vi "BonOMM-SAOMM.Test.vi"() -> ()   [LabVIEW 2011] (continued)
                                n2344 = local write "XReference"(w6163) -> ()
                                n2345 = local write "YReference"(w6164) -> ()
                                n2346 = Multiply(x=15.0, y=w6158) -> (x*y=w6156:dbl)
                                n2347 = Cosine(x=w6151) -> (cos(x)=w6155:dbl)
                                n2348 = Multiply(x=w6155, y=w6156) -> (x*y=w6154:dbl)
                                n2349 = property on="TableXYPos" class="XYGraph (strict)"("Cursor.Cursor Position:Cursor X"=w6154, "Cursor.Cursor Position:Cursor Y"=w6159) -> ()  [unwired: 2 in, 2 out]
                              }
                            }
                          }
                        }
                      }
                    }
                  }
                }
              }
              event "Centrage": Mouse Up {
                # "2 méthode en compétition ...\nPour l'instant on utilise Vrai"
                n2350 = event-data() -> ()  [unwired: 1 in, 7 out]
                n2351 = case shown="False" TRUE {
                  frame True {
                    # "YOffset"
                    # "XOffset"
                    # "RefY"
                    # "RefX"
                    # "ROIWidth"
                    # "ROIHeight"
                    # "Continuer?"
                    n2352 = stacked-sequence {
                      seq-local: [_ w6190 _ _ _] -> [_ _ w6214 w6240 _]
                      seq-local: [_ w6189 _ _ _] -> [_ _ _ _ _]
                      seq-local: [_ w6188 _ _ _] -> [_ _ _ _ _]
                      seq-local: [_ w6187 _ _ _] -> [_ _ _ _ _]
                      seq-local: [_ w6186 _ _ _] -> [_ _ _ _ _]
                      seq-local: [_ w6185 _ _ _] -> [_ _ _ _ _]
                      seq-local: [_ w6184 _ _ _] -> [_ _ _ _ _]
                      frame #0 {
                        n2353 = control-ref of="TERMINAL"() -> (w6182:refnum<vi>)
                        n2354 = control-ref of="Indicateur d'état"() -> (w6181:refnum<vi>)
                        n2355 = call "TERMINAL.vi"("Indicateur Refnum"=w6181, "Terminal Refnum"=w6182, "Indicateur d'état"="Lancement de la routine de centrage" ("string")) -> ()
                      }
                      frame #1 {
                        n2356 = local read "Integrating"() -> (w6197:bool)
                        n2357 = local read "SNR"() -> (w6193:dbl)
                        n2358 = local read "Servo"() -> (w6196:bool)
                        n2359 = local read "ROIXOffset"() -> (w6185:u16)
                        n2360 = local read "ROIYOffset"() -> (w6184:u16)
                        n2361 = local read "ROIHeight"() -> (w6188:u16)
                        n2362 = local read "ROIWidth"() -> (w6189:u16)
                        n2363 = local read "XROIRef"() -> (w6187:dbl)
                        n2364 = local read "YROIRef"() -> (w6186:dbl)
                        n2365 = Greater?(x=w6193, y=5.0) -> (0:w6191:bool)
                        n2366 = Not(x=w6196) -> (.not. x?=w6195:bool)
                        n2367 = Compound Arithmetic op=AND(w6191, w6197, w6195) -> (w6194:bool)
                        n2368 = case shown="True" w6194 {
                          tunnel: [FALSE w6200] -> w6190
                          frame False {
                            n2369 = One Button Dialog(message="Pour lancer la routine de centrage, assurez-vous que :\n  - la caméra fonctionne et est en acquisition\n  - une étoile est présente dans le champ (SNR>5)\n  - l'asservissement n'est pas actif") -> ()  [unwired: 1 in, 1 out]
                          }
                          frame True {
                            n2370 = Two Button Dialog(message="Désirez-vous lancer la routine de centrage ?\n(ceci déplacera les tables de translaions afin\nd'envoyer l'étoile au centre de la croisée)", 1:"Non" ("T button name (\"OK\")"), 2:"Oui" ("T button name (\"OK\")")) -> (T button?=w6200:bool)
                            n2371 = case shown="True" w6200 {
                              frame False {
                              }
                              frame True {
                                # "S'assure qu'on reçoit une nouvelle image ..."
                                n2372 = local read "LastImageID"() -> (w6204:u32)
                                n2373 = while {
                                tunnel: w6204 -> [w6212]
                                tunnel: [w6209] -> _
                                i -> [w6211]
                                stop <- w6210 stop-if-true
                                n2374 = local read "LastImageID"() -> (w6213:u32)
                                n2375 = Add(x=w6212, y=u32 1) -> (x+y=w6206:u32)
                                n2376 = Greater?(x=w6213, y=w6206) -> (0:w6209:bool)
                                n2377 = Wait Until Next ms Multiple(millisecond multiple=u32 100) -> ()  [unwired: 1 out]
                                n2378 = call "Max-iteration.vi"("i max"=600, "i act"=w6211, "Valeur entrante"=w6209) -> ("break ?"=w6210:bool)
                                }
                              }
                            }
                          }
                        }
                      }
                      frame #2 {
                        n2379 = case shown="True" w6214 {
                          frame False {
                          }
                          frame True {
                            n2380 = local read "GuiderAstrom"() -> (w6235:T4)
                            n2381 = local read "XCentroid"() -> (w6239:dbl)
                            n2382 = local read "YCentroid"() -> (w6238:dbl)
                            n2383 = local read "XReference"() -> (w6236:dbl)
                            n2384 = local read "YReference"() -> (w6237:dbl)
                            n2385 = local read "TableAstrom"() -> (w6230:T4)
                            n2386 = call "xy2ad.vi"("Y (px)"=w6238, "X (px)"=w6239, "Astrometry"=w6235) -> ("DEC (°)"=w6233:dbl, "RA (°)"=w6234:dbl)  [unwired: 5 in, 2 out]
                            n2387 = call "xy2ad.vi"("Y (px)"=w6237, "X (px)"=w6236, "Astrometry"=w6235) -> ("DEC (°)"=w6231:dbl, "RA (°)"=w6232:dbl)  [unwired: 5 in, 2 out]
                            n2388 = call "ad2xy.vi"("DEC"=w6233, "RA"=w6234, "Astrometry"=w6230) -> ("Y"=w6228:dbl, "X"=w6229:dbl)  [unwired: 6 in, 1 out]
                            n2389 = call "ad2xy.vi"("DEC"=w6231, "RA"=w6232, "Astrometry"=w6230) -> ("Y"=w6226:dbl, "X"=w6227:dbl)  [unwired: 6 in, 1 out]
                            n2390 = local read "Position Y"() -> (w6224:dbl)
                            n2391 = local read "Position X"() -> (w6225:dbl)
                            n2392 = formula code="cibX=tabX+(cenX-RefX);\ncibY=tabY+(cenY-RefY);"("cenX"=w6229, "tabX"=w6225, "tabY"=w6224, "cenY"=w6228, "RefX"=w6227, "RefY"=w6226) -> ("cibX"=w6223:dbl, "cibY"=w6222:dbl)
                            n2393 = local read "Position Z"() -> (w6221:dbl)
                            n2394 = local read "Table VRN"() -> (w6220:refnum<visa-resource-name>)
                            n2395 = local read "Table Error"() -> (w6218:errorcluster)
                            n2396 = local write "Cible X"(w6223) -> ()
                            n2397 = local write "Cible Y"(w6222) -> ()
                            n2398 = local write "Cible Z"(w6221) -> ()
                            n2399 = control-ref of="Table actif"() -> (w6215:refnum<vi>)
                            n2400 = call "Newmark-GotoAll.vi"("Table VRN IN"=w6220, "Bool Refnum"=w6215, "Notify?"=FALSE, "Error IN"=w6218, "Position X"=w6223, "Position Y"=w6222, "Position Z"=w6221) -> ("Table VRN OUT"=w6219:refnum<visa-resource-name>, "Error OUT"=w6217:errorcluster)  [unwired: 7 in]
                            n2401 = local write "Table VRN"(w6219) -> ()
                            n2402 = local write "Table Error"(w6217) -> ()
                          }
                        }
                      }
                      frame #3 {
                        # "Vérifie la cohérence des résultats obtenus ..."
                        n2403 = case shown="True" w6240 {
                          frame False {
                          }
                          frame True {
                            # "Au centre de la caméra ?"
                            # "Près du centre ?"
                            n2404 = local read "Position X"() -> (w6242:dbl)
                            n2405 = local read "Position Y"() -> (w6243:dbl)
                            n2406 = global read "Globals.vi" "EXIT"() -> (w6244:bool)
                            n2407 = In Range and Coerce(upper limit=500000.0, x=w6242, lower limit=450000.0 ("upper limit")) -> (In Range?=w6250:bool)  [unwired: 1 out]
                            n2408 = In Range and Coerce(upper limit=500000.0 ("lower limit"), x=w6243, lower limit=450000.0 ("upper limit")) -> (In Range?=w6251:bool)  [unwired: 1 out]
                            n2409 = local write "Indicateur d'état"("Centrage : vérification des résultats" ("Indicateur d'état")) -> ()
                            n2410 = Not(x=w6244) -> (.not. x?=w6241:bool)
                            n2411 = Compound Arithmetic op=AND(w6250, w6251, w6241) -> (w6252:bool)
                            n2412 = case shown="True" w6252 {
                              frame False {
                              }
                              frame True {
                                n2413 = Two Button Dialog(message="Voulez-vous utiliser ces valeurs\ncomme valeurs de centre (x,y) ?", 1:"Non" ("F button name (\"Cancel\")"), 2:"Oui" ("T button name (\"OK\")")) -> (T button?=w6253:bool)
                                n2414 = case shown="True" w6253 {
                                frame False {
                                }
                                frame True {
                                n2415 = stacked-sequence {
                                seq-local: [w6257 _] -> [_ w6263]
                                seq-local: [w6258 _] -> [_ w6264]
                                frame #0 {
                                n2416 = flat-sequence {
                                tunnel: [w6260] -> w6257
                                tunnel: [w6259] -> w6258
                                frame #0 {
                                n2417 = local read "Reference Y"() -> (w6260:dbl)
                                n2418 = local read "Reference X"() -> (w6259:dbl)
                                }
                                frame #1 {
                                n2419 = local read "Position Y"() -> (w6262:dbl)
                                n2420 = local write "Reference Y"(w6262) -> ()
                                n2421 = local read "Position X"() -> (w6261:dbl)
                                n2422 = local write "Reference X"(w6261) -> ()
                                }
                                }
                                }
                                frame #1 {
                                n2423 = Two Button Dialog(message="Voulez-vous vraiment utiliser ces \nvaleurs comme valeurs de centre (x,y) ?", 1:"Non" ("F button name (\"Cancel\")"), 2:"Oui" ("T button name (\"OK\")")) -> (T button?=w6265:bool)
                                n2424 = case shown="False" w6265 {
                                tunnel: w6264 -> [w6269 _]
                                tunnel: w6263 -> [w6270 _]
                                frame False {
                                n2425 = local write "Reference Y"(w6270) -> ()
                                n2426 = local write "Reference X"(w6269) -> ()
                                }
                                frame True {
                                }
                                }
                                }
                                }
                                }
                                }
                              }
                            }
                          }
                        }
                      }
                      frame #4 {
                        # "Pas certain que ce soit encore très utile ..."
                        n2427 = local write "Centrage_ready"(TRUE) -> ()
                        n2428 = global write "Globals.vi" "EXIT"(FALSE) -> ()
                        n2429 = local write "Indicateur d'état"("Centrage : fin de la routine" ("Indicateur d'état")) -> ()
                      }
                    }
                  }
                  frame False {
                    # "YOffset"
                    # "XOffset"
                    # "RefY"
                    # "RefX"
                    # "ROIWidth"
                    # "ROIHeight"
                    # "Continuer?"
                    n2430 = stacked-sequence {
                      seq-local: [_ w6283 _ _ _ _] -> [_ _ w6338 w6376 _ _]
                      seq-local: [_ w6282 _ _ _ _] -> [_ _ _ _ w6416 _]
                      seq-local: [_ w6281 _ _ _ _] -> [_ _ _ _ w6415 _]
                      seq-local: [_ w6280 _ _ _ _] -> [_ _ _ _ w6410 _]
                      seq-local: [_ w6279 _ _ _ _] -> [_ _ _ _ w6409 _]
                      seq-local: [_ w6278 _ _ _ _] -> [_ _ _ _ w6408 _]
                      seq-local: [_ w6277 _ _ _ _] -> [_ _ _ _ w6407 _]
                      frame #0 {
                        n2431 = control-ref of="TERMINAL"() -> (w6275:refnum<vi>)
                        n2432 = control-ref of="Indicateur d'état"() -> (w6274:refnum<vi>)
                        n2433 = call "TERMINAL.vi"("Indicateur Refnum"=w6274, "Terminal Refnum"=w6275, "Indicateur d'état"="Lancement de la routine de centrage" ("string")) -> ()
                      }
                      frame #1 {
                        n2434 = local read "Integrating"() -> (w6290:bool)
                        n2435 = local read "SNR"() -> (w6286:dbl)
                        n2436 = local read "Servo"() -> (w6289:bool)
                        n2437 = local read "ROIXOffset"() -> (w6278:u16)
                        n2438 = local read "ROIYOffset"() -> (w6277:u16)
                        n2439 = local read "ROIHeight"() -> (w6281:u16)
                        n2440 = local read "ROIWidth"() -> (w6282:u16)
                        n2441 = local read "XROIRef"() -> (w6280:dbl)
                        n2442 = local read "YROIRef"() -> (w6279:dbl)
                        n2443 = Greater?(x=w6286, y=5.0) -> (0:w6284:bool)
                        n2444 = Not(x=w6289) -> (.not. x?=w6288:bool)
                        n2445 = Compound Arithmetic op=AND(w6284, w6290, w6288) -> (w6287:bool)
                        n2446 = case shown="True" w6287 {
                          tunnel: [FALSE w6293] -> w6283
                          frame False {
                            n2447 = One Button Dialog(message="Pour lancer la routine de centrage, assurez-vous que :\n  - la caméra fonctionne et est en acquisition\n  - une étoile est présente dans le champ (SNR>5)\n  - l'asservissement n'est pas actif") -> ()  [unwired: 1 in, 1 out]
                          }
                          frame True {
                            n2448 = Two Button Dialog(message="Désirez-vous lancer la routine de centrage ?\n(ceci déplacera les tables de translaions afin\nd'envoyer l'étoile au centre de la caméra)", 1:"Non" ("T button name (\"OK\")"), 2:"Oui" ("T button name (\"OK\")")) -> (T button?=w6294:bool)
                            n2449 = case shown="True" w6294 {
                              selector: w6294 -> [w6298 _]
                              tunnel: [w6298 w6313] -> w6293
                              frame False {
                              }
                              frame True {
                                # "Remplacer par\naucune erreur\n(PrAMS)"
                                n2450 = local read "ImageHeight"() -> (w6299:u16)
                                n2451 = local read "ImageWidth"() -> (w6300:u16)
                                n2452 = local read "PrAMS VRN"() -> (w6337:refnum<visa-resource-name>)
                                n2453 = local read "PrAMS Error"() -> (w6336:errorcluster)
                                n2454 = local read "MessageType"() -> (w6322:cluster{string[], u32[]})
                                n2455 = control-ref of="PrAMS-ACK"() -> (w6316:refnum<vi>)
                                n2456 = control-ref of="PrAMS actif"() -> (w6317:refnum<vi>)
                                n2457 = local read "Signature"() -> (w6323:u32)
                                n2458 = call-poly "SAOMM-Num2littleEndian.vi"("Number"=u16 0) -> ("LiitleEndianedData"=w6319:u8[])  [unwired: 14 in]
                                n2459 = call-poly "SAOMM-Num2littleEndian.vi"("Number"=u16 0) -> ("LiitleEndianedData"=w6318:u8[])  [unwired: 14 in]
                                n2460 = call-poly "SAOMM-Num2littleEndian.vi"("Number"=w6300) -> ("LiitleEndianedData"=w6311:u8[])  [unwired: 14 in]
                                n2461 = call-poly "SAOMM-Num2littleEndian.vi"("Number"=w6299) -> ("LiitleEndianedData"=w6309:u8[])  [unwired: 14 in]
                                n2462 = To Double Precision Float(number=w6300) -> (double precision float=w6304:dbl)
                                n2463 = To Double Precision Float(number=w6299) -> (double precision float=w6302:dbl)
                                n2464 = call "SAOMM-SendSET.vi"("PRAMMS-COMM IN"=w6337, "Active Refnum"=w6317, "PrAMS-ACK"=w6316, "Signature"=w6323, "Error IN"=w6336, "MessageType"=w6322, "Active SET"="emtSetROIXOffset", "Value (little endianed byte array)"=w6319) -> ("PRAMMS-COMM OUT"=w6335:refnum<visa-resource-name>, "Error OUT"=w6332:errorcluster)  [unwired: 4 in, 2 out]
                                n2465 = expression code="x/2"(w6304) -> (w6303:dbl)
                                n2466 = expression code="x/2"(w6302) -> (w6301:dbl)
                                n2467 = call "SAOMM-SendSET.vi"("PRAMMS-COMM IN"=w6335, "Active Refnum"=w6317, "PrAMS-ACK"=w6316, "Signature"=w6323, "Error IN"=w6332, "MessageType"=w6322, "Active SET"="emtSetROIYOffset", "Value (little endianed byte array)"=w6318) -> ("PRAMMS-COMM OUT"=w6334:refnum<visa-resource-name>, "Error OUT"=w6331:errorcluster)  [unwired: 4 in, 2 out]
                                n2468 = call-poly "SAOMM-Num2littleEndian.vi"("Number"=w6303) -> ("LiitleEndianedData"=w6308:u8[])  [unwired: 14 in]
                                n2469 = call-poly "SAOMM-Num2littleEndian.vi"("Number"=w6301) -> ("LiitleEndianedData"=w6305:u8[])  [unwired: 14 in]
                                n2470 = call "SAOMM-SendSET.vi"("PRAMMS-COMM IN"=w6334, "Active Refnum"=w6317, "PrAMS-ACK"=w6316, "Signature"=w6323, "Error IN"=w6331, "MessageType"=w6322, "Active SET"="emtSetROIHeight", "Value (little endianed byte array)"=w6311) -> ("PRAMMS-COMM OUT"=w6333:refnum<visa-resource-name>, "Error OUT"=w6330:errorcluster)  [unwired: 4 in, 2 out]
                                n2471 = call "SAOMM-SendSET.vi"("PRAMMS-COMM IN"=w6333, "Active Refnum"=w6317, "PrAMS-ACK"=w6316, "Signature"=w6323, "Error IN"=w6330, "MessageType"=w6322, "Active SET"="emtSetROIWidth", "Value (little endianed byte array)"=w6309) -> ("PRAMMS-COMM OUT"=w6325:refnum<visa-resource-name>, "Error OUT"=w6324:errorcluster)  [unwired: 4 in, 2 out]
                                n2472 = call "SAOMM-SendSET.vi"("PRAMMS-COMM IN"=w6325, "Active Refnum"=w6317, "PrAMS-ACK"=w6316, "Signature"=w6323, "Error IN"=w6324, "MessageType"=w6322, "Active SET"="emtSetROIXReferencePoint", "Value (little endianed byte array)"=w6308) -> ("PRAMMS-COMM OUT"=w6326:refnum<visa-resource-name>, "Error OUT"=w6327:errorcluster)  [unwired: 4 in, 2 out]
                                n2473 = call "SAOMM-SendSET.vi"("PRAMMS-COMM IN"=w6326, "Active Refnum"=w6317, "PrAMS-ACK"=w6316, "Signature"=w6323, "Error IN"=w6327, "MessageType"=w6322, "Active SET"="emtSetROIYReferencePoint", "Value (little endianed byte array)"=w6305) -> ("Error"=w6314:bool, "Error OUT"=w6315:errorcluster)  [unwired: 4 in, 2 out]
                                n2474 = local write "PrAMS Error"(w6315) -> ()
                                n2475 = Not(x=w6314) -> (.not. x?=w6313:bool)
                              }
                            }
                          }
                        }
                      }
                      frame #2 {
                        n2476 = case shown="True" w6338 {
                          frame False {
                          }
                          frame True {
                            # "S'assure qu'on reçoit une nouvelle image ..."
                            n2477 = local read "LastImageID"() -> (w6340:u32)
                            n2478 = while {
                              tunnel: w6340 -> [w6374]
                              tunnel: [w6371] -> w6339
                              i -> [w6373]
                              stop <- w6372 stop-if-true
                              n2479 = local read "LastImageID"() -> (w6375:u32)
                              n2480 = Add(x=w6374, y=u32 5) -> (x+y=w6368:u32)
                              n2481 = Greater?(x=w6375, y=w6368) -> (0:w6371:bool)
                              n2482 = Wait Until Next ms Multiple(millisecond multiple=u32 100) -> ()  [unwired: 1 out]
                              n2483 = call "Max-iteration.vi"("i max"=600, "i act"=w6373, "Valeur entrante"=w6371) -> ("break ?"=w6372:bool)
                            }
                            n2484 = case shown="True" w6339 {
                              frame False {
                              }
                              frame True {
                                # "Direction à confirmer ..."
                                n2485 = local read "ImageWidth"() -> (w6345:u16)
                                n2486 = local read "ImageHeight"() -> (w6344:u16)
                                n2487 = local read "Binning"() -> (w6343:u16)
                                n2488 = To Double Precision Float(number=w6345) -> (double precision float=w6347:dbl)
                                n2489 = To Double Precision Float(number=w6344) -> (double precision float=w6346:dbl)
                                n2490 = expression code="x/2"(w6347) -> (w6341:dbl)
                                n2491 = expression code="x/2"(w6346) -> (w6342:dbl)
                                n2492 = local read "XCentroid"() -> (w6353:dbl)
                                n2493 = local read "PixScale1"() -> (w6357:dbl)
                                n2494 = local read "PixScale2"() -> (w6356:dbl)
                                n2495 = local read "YCentroid"() -> (w6354:dbl)
                                n2496 = local read "arcsec/pulse"() -> (w6348:dbl)
                                n2497 = To Double Precision Float(number=w6343) -> (double precision float=w6355:dbl)
                                n2498 = formula code="deltax=cenx-refx;\ncorrx=deltax*(pxscl1*bin)/tabscl;\ndeltay=ceny-refy;\ncorry=deltay*(pxscl2*bin)/tabscl;"("pxscl1"=w6357, "pxscl2"=w6356, "bin"=w6355, "refx"=w6341, "refy"=w6342, "cenx"=w6353, "ceny"=w6354, "tabscl"=w6348) -> ("corrx"=w6349:dbl, "corry"=w6350:dbl)  [unwired: 2 out]
                                n2499 = local read "Position X"() -> (w6352:dbl)
                                n2500 = local read "Position Y"() -> (w6351:dbl)
                                n2501 = local read "Position Z"() -> (w6360:dbl)
                                n2502 = Subtract(x=w6351, y=w6350) -> (x-y=w6359:dbl)
                                n2503 = Subtract(x=w6352, y=w6349) -> (x-y=w6358:dbl)
                                n2504 = local write "Cible X"(w6358) -> ()
                                n2505 = local write "Cible Y"(w6359) -> ()
                                n2506 = local write "Cible Z"(w6360) -> ()
                                n2507 = local read "Table VRN"() -> (w6366:refnum<visa-resource-name>)
                                n2508 = local read "Table Error"() -> (w6364:errorcluster)
                                n2509 = control-ref of="Table actif"() -> (w6361:refnum<vi>)
                                n2510 = call "Newmark-GotoAll.vi"("Table VRN IN"=w6366, "Bool Refnum"=w6361, "Notify?"=FALSE, "Error IN"=w6364, "Position X"=w6358, "Position Y"=w6359, "Position Z"=w6360) -> ("Table VRN OUT"=w6365:refnum<visa-resource-name>, "Error OUT"=w6363:errorcluster)  [unwired: 7 in]
                                n2511 = local write "Table VRN"(w6365) -> ()
                                n2512 = local write "Table Error"(w6363) -> ()
                              }
                            }
                          }
                        }
                      }
                      frame #3 {
                        # "Vérifie la cohérence des résultats obtenus ..."
                        n2513 = case shown="True" w6376 {
                          frame False {
                          }
                          frame True {
                            n2514 = local read "Position X"() -> (w6378:dbl)
                            n2515 = local read "Position Y"() -> (w6379:dbl)
                            n2516 = In Range and Coerce(upper limit=500000.0, x=w6378, lower limit=450000.0 ("upper limit")) -> (In Range?=w6386:bool)  [unwired: 1 out]
                            n2517 = In Range and Coerce(upper limit=500000.0 ("lower limit"), x=w6379, lower limit=450000.0 ("upper limit")) -> (In Range?=w6387:bool)  [unwired: 1 out]
                            n2518 = local write "Indicateur d'état"("Centrage : vérification des résultats" ("Indicateur d'état")) -> ()
                            n2519 = global read "Globals.vi" "EXIT"() -> (w6380:bool)
                            n2520 = Not(x=w6380) -> (.not. x?=w6377:bool)
                            n2521 = Compound Arithmetic op=AND(w6386, w6387, w6377) -> (w6388:bool)
                            n2522 = case shown="True" w6388 {
                              frame False {
                              }
                              frame True {
                                n2523 = Two Button Dialog(message="Voulez-vous utiliser ces valeurs\ncomme valeurs de centre (x,y)", 1:"Non" ("F button name (\"Cancel\")"), 2:"Oui" ("T button name (\"OK\")")) -> (T button?=w6389:bool)
                                n2524 = case shown="True" w6389 {
                                frame False {
                                }
                                frame True {
                                n2525 = stacked-sequence {
                                seq-local: [w6393 _] -> [_ w6399]
                                seq-local: [w6394 _] -> [_ w6400]
                                frame #0 {
                                n2526 = flat-sequence {
                                tunnel: [w6396] -> w6393
                                tunnel: [w6395] -> w6394
                                frame #0 {
                                n2527 = local read "Reference Y"() -> (w6396:dbl)
                                n2528 = local read "Reference X"() -> (w6395:dbl)
                                }
                                frame #1 {
                                n2529 = local read "Position Y"() -> (w6398:dbl)
                                n2530 = local write "Reference Y"(w6398) -> ()
                                n2531 = local read "Position X"() -> (w6397:dbl)
                                n2532 = local write "Reference X"(w6397) -> ()
                                }
                                }
                                }
                                frame #1 {
                                n2533 = Two Button Dialog(message="Voulez-vous vraiment utiliser ces \nvaleurs comme valeurs de centre (x,y)", 1:"Non" ("F button name (\"Cancel\")"), 2:"Oui" ("T button name (\"OK\")")) -> (T button?=w6401:bool)
                                n2534 = case shown="False" w6401 {
                                tunnel: w6400 -> [w6405 _]
                                tunnel: w6399 -> [w6406 _]
                                frame False {
                                n2535 = local write "Reference Y"(w6406) -> ()
                                n2536 = local write "Reference X"(w6405) -> ()
                                }
                                frame True {
                                }
                                }
                                }
                                }
                                }
                                }
                              }
                            }
                          }
                        }
                      }
                      frame #4 {
                        n2537 = local read "PrAMS VRN"() -> (w6441:refnum<visa-resource-name>)
                        n2538 = local read "PrAMS Error"() -> (w6440:errorcluster)
                        n2539 = local read "MessageType"() -> (w6426:cluster{string[], u32[]})
                        n2540 = control-ref of="PrAMS-ACK"() -> (w6418:refnum<vi>)
                        n2541 = control-ref of="PrAMS actif"() -> (w6419:refnum<vi>)
                        n2542 = local read "Signature"() -> (w6429:u32)
                        n2543 = call-poly "SAOMM-Num2littleEndian.vi"("Number"=w6416) -> ("LiitleEndianedData"=w6425:u8[])  [unwired: 14 in]
                        n2544 = call-poly "SAOMM-Num2littleEndian.vi"("Number"=w6415) -> ("LiitleEndianedData"=w6424:u8[])  [unwired: 14 in]
                        n2545 = call-poly "SAOMM-Num2littleEndian.vi"("Number"=w6410) -> ("LiitleEndianedData"=w6423:u8[])  [unwired: 14 in]
                        n2546 = call-poly "SAOMM-Num2littleEndian.vi"("Number"=w6409) -> ("LiitleEndianedData"=w6422:u8[])  [unwired: 14 in]
                        n2547 = call-poly "SAOMM-Num2littleEndian.vi"("Number"=w6408) -> ("LiitleEndianedData"=w6421:u8[])  [unwired: 14 in]
                        n2548 = call-poly "SAOMM-Num2littleEndian.vi"("Number"=w6407) -> ("LiitleEndianedData"=w6420:u8[])  [unwired: 14 in]
                        n2549 = call "SAOMM-SendSET.vi"("PRAMMS-COMM IN"=w6441, "Active Refnum"=w6419, "PrAMS-ACK"=w6418, "Signature"=w6429, "Error IN"=w6440, "MessageType"=w6426, "Active SET"="emtSetROIHeight", "Value (little endianed byte array)"=w6425) -> ("PRAMMS-COMM OUT"=w6439:refnum<visa-resource-name>, "Error OUT"=w6436:errorcluster)  [unwired: 4 in, 2 out]
                        n2550 = call "SAOMM-SendSET.vi"("PRAMMS-COMM IN"=w6439, "Active Refnum"=w6419, "PrAMS-ACK"=w6418, "Signature"=w6429, "Error IN"=w6436, "MessageType"=w6426, "Active SET"="emtSetROIWidth", "Value (little endianed byte array)"=w6424) -> ("PRAMMS-COMM OUT"=w6438:refnum<visa-resource-name>, "Error OUT"=w6435:errorcluster)  [unwired: 4 in, 2 out]
                        n2551 = call "SAOMM-SendSET.vi"("PRAMMS-COMM IN"=w6438, "Active Refnum"=w6419, "PrAMS-ACK"=w6418, "Signature"=w6429, "Error IN"=w6435, "MessageType"=w6426, "Active SET"="emtSetROIXReferencePoint", "Value (little endianed byte array)"=w6423) -> ("PRAMMS-COMM OUT"=w6437:refnum<visa-resource-name>, "Error OUT"=w6434:errorcluster)  [unwired: 4 in, 2 out]
                        n2552 = call "SAOMM-SendSET.vi"("PRAMMS-COMM IN"=w6437, "Active Refnum"=w6419, "PrAMS-ACK"=w6418, "Signature"=w6429, "Error IN"=w6434, "MessageType"=w6426, "Active SET"="emtSetROIYReferencePoint", "Value (little endianed byte array)"=w6422) -> ("PRAMMS-COMM OUT"=w6431:refnum<visa-resource-name>, "Error OUT"=w6430:errorcluster)  [unwired: 4 in, 2 out]
                        n2553 = call "SAOMM-SendSET.vi"("PRAMMS-COMM IN"=w6431, "Active Refnum"=w6419, "PrAMS-ACK"=w6418, "Signature"=w6429, "Error IN"=w6430, "MessageType"=w6426, "Active SET"="emtSetROIXOffset", "Value (little endianed byte array)"=w6421) -> ("PRAMMS-COMM OUT"=w6432:refnum<visa-resource-name>, "Error OUT"=w6433:errorcluster)  [unwired: 4 in, 2 out]
                        n2554 = call "SAOMM-SendSET.vi"("PRAMMS-COMM IN"=w6432, "Active Refnum"=w6419, "PrAMS-ACK"=w6418, "Signature"=w6429, "Error IN"=w6433, "MessageType"=w6426, "Active SET"="emtSetROIYOffset", "Value (little endianed byte array)"=w6420) -> ("Error OUT"=w6417:errorcluster)  [unwired: 4 in, 3 out]
                        n2555 = local write "PrAMS Error"(w6417) -> ()
                      }
                      frame #5 {
                        # "Pas certain que ce soit encore très utile ..."
                        n2556 = local write "Centrage_ready"(TRUE) -> ()
                        n2557 = global write "Globals.vi" "EXIT"(FALSE) -> ()
                        n2558 = local write "Indicateur d'état"("Centrage : fin de la routine" ("Indicateur d'état")) -> ()
                      }
                    }
                  }
                }
                n2559 = flat-sequence {
                  tunnel: [FALSE ("CentrageLed")] -> w6178
                  frame #0 {
                    "Centrage_ready" <- FALSE
                  }
                  frame #1 {
                    n2560 = while {
                      stop <- w6447 stop-if-true
                      n2561 = local read "CentrageLed"() -> (w6449:bool)
                      n2562 = Wait (ms)(milliseconds to wait=u32 250) -> ()  [unwired: 1 out]
                      n2563 = Not(x=w6449) -> (.not. x?=→"CentrageLed":bool)
                      n2564 = local read "Centrage_ready"() -> (w6447:bool)
                    }
                  }
                }
                n2565 = global write "Globals.vi" "EXIT"(FALSE ("Visible")) -> ()
                n2566 = local write "CentrageLed"(w6178) -> ()
              }
              event "ST+", "ST-": Value Change {
                n2567 = event-data() -> ()  [unwired: 1 in, 6 out]
                n2568 = Build Array("ST+", "ST-") -> (w6453:bool[])
                n2569 = Boolean Array To Number(Boolean array=w6453) -> (number=w6452:u32)
                n2570 = local read "MC-BonOMM VRN"() -> (w6451:refnum<visa-resource-name>)
                n2571 = case shown="2" w6452 {
                  tunnel: w6451 -> [_ w6458 w6478]
                  frame 0, Default {
                  }
                  frame 2 {
                    n2572 = call "MC-BonOMM_talker.vi"("MC-BonOMM VRN"=w6458, "Commande"="-" ("write buffer"), "Timeout (ms)"=1000, "answer=command?"=TRUE) -> ("ok ?"=w6456:bool)  [unwired: 1 in, 1 out]
                    n2573 = case shown="True" w6456 {
                      tunnel: w6458 -> [w6461 w6472]
                      frame False {
                        n2574 = One Button Dialog(message="Erreur lors de la commande de déplacement", button name ("OK")="Ok ?!?") -> ()  [unwired: 1 out]
                        n2575 = call "MC-BonOMM_talker.vi"("MC-BonOMM VRN"=w6461, "Commande"="s" ("write buffer"), "Timeout (ms)"=1000, "answer=command?"=TRUE) -> ()  [unwired: 1 in, 2 out]
                      }
                      frame True {
                        n2576 = while {
                          tunnel: w6472 -> [w6474]
                          tunnel: [w6474] -> w6471
                          stop <- w6473 continue-if-true
                          n2577 = local read "ST-"() -> (w6473:bool)
                          n2578 = Wait (ms)(milliseconds to wait=u32 50) -> ()  [unwired: 1 out]
                        }
                        n2579 = call "MC-BonOMM_talker.vi"("MC-BonOMM VRN"=w6471, "Commande"="s" ("write buffer"), "Timeout (ms)"=1000, "answer=command?"=TRUE) -> ("ok ?"=w6467:bool)  [unwired: 1 in, 1 out]
                        n2580 = local write "MC_connect"(w6467) -> ()
                      }
                    }
                    n2581 = local write "MC_connect"(w6456) -> ()
                  }
                  frame 1 {
                    n2582 = call "MC-BonOMM_talker.vi"("MC-BonOMM VRN"=w6478, "Commande"="+" ("write buffer"), "Timeout (ms)"=1000, "answer=command?"=TRUE) -> ("ok ?"=w6476:bool)  [unwired: 1 in, 1 out]
                    n2583 = case shown="True" w6476 {
                      tunnel: w6478 -> [w6482 w6493]
                      frame False {
                        n2584 = One Button Dialog(message="Erreur lors de la commande de déplacement", button name ("OK")="Ok ?!?") -> ()  [unwired: 1 out]
                        n2585 = call "MC-BonOMM_talker.vi"("MC-BonOMM VRN"=w6482, "Commande"="s" ("write buffer"), "Timeout (ms)"=1000, "answer=command?"=TRUE) -> ("ok ?"=w6481:bool)  [unwired: 1 in, 1 out]
                        n2586 = local write "MC_connect"(w6481) -> ()
                      }
                      frame True {
                        n2587 = while {
                          tunnel: w6493 -> [w6495]
                          tunnel: [w6495] -> w6492
                          stop <- w6494 continue-if-true
                          n2588 = local read "ST+"() -> (w6494:bool)
                          n2589 = Wait (ms)(milliseconds to wait=u32 50) -> ()  [unwired: 1 out]
                        }
                        n2590 = call "MC-BonOMM_talker.vi"("MC-BonOMM VRN"=w6492, "Commande"="s" ("write buffer"), "Timeout (ms)"=1000, "answer=command?"=TRUE) -> ("ok ?"=w6488:bool)  [unwired: 1 in, 1 out]
                        n2591 = local write "MC_connect"(w6488) -> ()
                      }
                    }
                    n2592 = local write "MC_connect"(w6476) -> ()
                  }
                }
              }
              event "Ajust z to tel": Value Change {
                n2593 = event-data() -> ()  [unwired: 1 in, 6 out]
                n2594 = local read "Foyer"() -> (w6497:dbl)
                n2595 = case shown="True" "Ajust z to tel" {
                  tunnel: w6497 -> [_ w6513]
                  frame False {
                  }
                  frame True {
                    n2596 = local read "k0_focus"() -> (w6509:dbl)
                    n2597 = local read "k1_focus"() -> (w6508:dbl)
                    n2598 = formula code="foyersonde=foyertel*k1+k0;"("foyertel"=w6513, "k0"=w6509, "k1"=w6508) -> ("foyersonde"=w6500:dbl)
                    n2599 = local read "CentreTel X"() -> (w6507:dbl)
                    n2600 = local read "CentreTel Y"() -> (w6506:dbl)
                    n2601 = local read "Position X"() -> (w6502:dbl)
                    n2602 = local read "Position Y"() -> (w6501:dbl)
                    n2603 = local read "a1_focus"() -> (w6505:dbl)
                    n2604 = local read "a2_focus"() -> (w6504:dbl)
                    n2605 = local read "a3_focus"() -> (w6503:dbl)
                    n2606 = control-ref of="TERMINAL"() -> (w6511:refnum<vi>)
                    n2607 = control-ref of="Indicateur d'état"() -> (w6512:refnum<vi>)
                    n2608 = call "Calc_focus.vi"("Pos X"=w6502, "a0"=w6500, "Pos Y"=w6501, "Cen X"=w6507, "Cen Y"=w6506, "a1"=w6505, "a2"=w6504, "a3"=w6503) -> ("Foyer"=w6499:dbl)  [unwired: 6 in, 1 out]
                    n2609 = call "TERMINAL.vi"("Indicateur Refnum"=w6512, "Terminal Refnum"=w6511, "Indicateur d'état"="Ajustement automatique du foyer de la caméra de guidage") -> ()
                    n2610 = local write "FoyerAuCentre"(w6500) -> ()
                    n2611 = property on="FoyerTable" class="DigNum (strict)"("Val(Sgnl)"=w6499) -> ()  [unwired: 2 in, 2 out]
                  }
                }
              }
              event "Foyer+", "Foyer-": Mouse Down {
                n2612 = event-data() -> ()  [unwired: 1 in, 8 out]
                n2613 = Or(x="Foyer+", y="Foyer-") -> (x .or. y?=w6515:bool)
                n2614 = case shown="True" w6515 {
                  tunnel: "Foyer+" -> [_ w6539]
                  frame False {
                  }
                  frame True {
                    w6525 = "AZ" ("StageTag")
                    n2615 = local read "vitesse focus"() -> (w6538:dbl)
                    n2616 = control-ref of="TERMINAL"() -> (w6530:refnum<vi>)
                    n2617 = control-ref of="Indicateur d'état"() -> (w6529:refnum<vi>)
                    n2618 = Negate(x=w6538) -> (-x=w6537:dbl)
                    n2619 = local write "Focusing"(TRUE ("Focusing")) -> ()
                    n2620 = Select(t=w6538, s=w6539, f=w6537) -> (s? t:f=w6524:dbl)
                    n2621 = local read "Table VRN"() -> (w6536:refnum<visa-resource-name>)
                    n2622 = local read "Table Error"() -> (w6535:errorcluster)
                    n2623 = call "TERMINAL.vi"("Indicateur Refnum"=w6529, "Terminal Refnum"=w6530, "Indicateur d'état"="Modification du foyer \"au centre\" de la caméra de guidage") -> ()
                    n2624 = control-ref of="Table actif"() -> (w6532:refnum<vi>)
                    n2625 = call "Newmark-Jog.vi"("Table VRN IN"=w6536, "StageTag"=w6525, "Bool Refnum"=w6532, "Error IN"=w6535, "Velocity"=w6524) -> ("Table VRN OUT"=w6533:refnum<visa-resource-name>, "Error OUT"=w6534:errorcluster)  [unwired: 9 in]
                    n2626 = flat-sequence {
                      tunnel: w6533 -> [w6543]
                      tunnel: w6534 -> [w6542]
                      tunnel: [w6543] -> w6528
                      tunnel: [w6542] -> w6527
                      tunnel: [w6541] -> w6526
                      tunnel: w6525 -> [w6541]
                      tunnel: [w6540] -> _
                      tunnel: w6527 -> [w6555]
                      tunnel: w6528 -> [w6556]
                      tunnel: [w6553] -> w6523
                      tunnel: [w6552] -> w6521
                      tunnel: [w6554] -> w6519
                      tunnel: w6526 -> [w6554]
                      tunnel: w6523 -> [w6560]
                      tunnel: [w6560] -> w6522
                      tunnel: w6521 -> [w6559]
                      tunnel: [w6559] -> w6520
                      tunnel: w6519 -> [w6558]
                      tunnel: [w6558] -> w6518
                      tunnel: w6522 -> [w6571]
                      tunnel: w6520 -> [w6570]
                      tunnel: w6518 -> [w6569]
                      frame #0 {
                        n2627 = while {
                          tunnel: [w6544] -> w6540
                          stop <- w6546 continue-if-true
                          n2628 = local read "Exceptions"() -> (w6545:T3)
                          n2629 = local read "Foyer-"() -> (w6549:bool)
                          n2630 = local read "Foyer+"() -> (w6550:bool)
                          n2631 = Unbundle By Name(w6545) -> ("Overtravel"=w6544:bool)
                          n2632 = Or(x=w6550, y=w6549) -> (x .or. y?=w6547:bool)
                          n2633 = Wait (ms)(milliseconds to wait=u32 100) -> ()  [unwired: 1 out]
                          n2634 = Not(x=w6544) -> (.not. x?=w6548:bool)
                          n2635 = And(x=w6547, y=w6548) -> (x .and. y?=w6546:bool)
                        }
                      }
                      frame #1 {
                        n2636 = control-ref of="Table actif"() -> (w6557:refnum<vi>)
                        n2637 = call "Newmark-Stop.vi"("Table VRN IN"=w6556, "Bool Refnum"=w6557, "Error IN"=w6555) -> ("Table VRN OUT"=w6553:refnum<visa-resource-name>, "Error OUT"=w6552:errorcluster)  [unwired: 11 in]
                      }
                      frame #2 {
                        n2638 = while {
                          stop <- w6562 continue-if-true
                          n2639 = local read "MovingZ"() -> (w6562:bool)
                          n2640 = Wait (ms)(milliseconds to wait=u32 100) -> ()  [unwired: 1 out]
                        }
                      }
                      frame #3 {
                        n2641 = local read "vitesse rapide"() -> (w6566:dbl)
                        n2642 = local read "vitesse lente"() -> (w6567:dbl)
                        n2643 = local read "accelleration"() -> (w6565:dbl)
                        n2644 = control-ref of="Table actif"() -> (w6568:refnum<vi>)
                        n2645 = call "Newmark-SetSpeed.vi"("Table VRN"=w6571, "StageTAG"=w6569, "Bool Refnum"=w6568, "Error IN"=w6570, "Vitesse Lente"=w6567, "Vitesse Rapide"=w6566, "Accélération"=w6565) -> ("Table VRN OUT"=w6564:refnum<visa-resource-name>, "Error OUT"=w6563:errorcluster)  [unwired: 6 in, 1 out]
                        n2646 = local write "Table VRN"(w6564) -> ()
                        n2647 = local write "Table Error"(w6563) -> ()
                      }
                    }
                  }
                }
              }
              event "FoyerTable": Value Change {
                n2648 = event-data() -> ("NewVal"=w6574:dbl)  [unwired: 1 in, 5 out]
                n2649 = local write "Cible Z"(w6574) -> ()
                n2650 = local read "Table VRN"() -> (w6581:refnum<visa-resource-name>)
                n2651 = local read "Table Error"() -> (w6579:errorcluster)
                n2652 = control-ref of="Table actif"() -> (w6577:refnum<vi>)
                n2653 = local write "CorrectZ"(TRUE ("CorrectZ")) -> ()
                n2654 = call "Newmark-GotoOne.vi"("Table VRN IN"=w6581, "Bool Refnum"=w6577, "StageTAG"="AZ", "Notify?"=FALSE, "Error IN"=w6579, "Position"=w6574) -> ("Table VRN OUT"=w6580:refnum<visa-resource-name>, "Error OUT"=w6578:errorcluster)  [unwired: 8 in]
                n2655 = local write "Focusing"(TRUE ("Focusing")) -> ()
                n2656 = local write "Table VRN"(w6580) -> ()
                n2657 = local write "Table Error"(w6578) -> ()
                n2658 = Unbundle By Name(w6578) -> ("status"=w6582:bool)
                n2659 = Not(x=w6582) -> ()  [unwired: 1 out]
              }
              event "ApplyCorrection": Value Change {
                n2660 = event-data() -> ()  [unwired: 1 in, 6 out]
                n2661 = local read "ApplyCorrection"() -> (w6583:bool)
                n2662 = case shown="True" w6583 {
                  frame False {
                  }
                  frame True {
                    n2663 = local read "Cible X"() -> (w6589:dbl)
                    n2664 = local read "Position X"() -> (w6586:dbl)
                    n2665 = local read "Cible Y"() -> (w6587:dbl)
                    n2666 = local read "Position Y"() -> (w6588:dbl)
                    n2667 = local read "Cible Z"() -> (w6591:dbl)
                    n2668 = local read "Position Z"() -> (w6590:dbl)
                    n2669 = Subtract(x=w6587, y=w6588) -> (x-y=w6584:dbl)
                    n2670 = Subtract(x=w6589, y=w6586) -> (x-y=w6585:dbl)
                    n2671 = Subtract(x=w6591, y=w6590) -> (x-y=w6595:dbl)
                    n2672 = local read "Table Error"() -> (w6599:errorcluster)
                    n2673 = local read "Table VRN"() -> (w6600:refnum<visa-resource-name>)
                    n2674 = Build Array(w6585, w6584, w6595) -> (w6594:dbl[])
                    n2675 = control-ref of="Table actif"() -> (w6598:refnum<vi>)
                    n2676 = local write "ApplyCorrection"(FALSE ("Correct")) -> ()
                    n2677 = call "Newmark-CorrectPosition.vi"("Table VRN IN"=w6600, "Bool Refnum"=w6598, "Error IN"=w6599, "StageTags"=string[] ["AX", "AY", "AZ"], "Corrections"=w6594) -> ("Table VRN OUT"=w6597:refnum<visa-resource-name>, "Error OUT"=w6596:errorcluster)  [unwired: 8 in, 1 out]
                    n2678 = local write "Table VRN"(w6597) -> ()
                    n2679 = local write "Table Error"(w6596) -> ()
                  }
                }
              }
              event "YReference", "XReference": Value Change {
                n2680 = event-data() -> ()  [unwired: 1 in, 6 out]
                n2681 = control-ref of="ImgArray"() -> (w6609:refnum<vi>)
                n2682 = local read "ROIHeight"() -> (w6607:u16)
                n2683 = local read "ROIWidth"() -> (w6608:u16)
                n2684 = call "SAOMM-Cursor2ROI.vi"("ImgRef"=w6609, "CursorX"="XReference", "CursorY"="YReference", "ROIWidth"=w6608, "ROIHeight"=w6607) -> ("ROIXOffset"=w6606:u16, "ROIYOffset"=w6605:u16)  [unwired: 7 in, 2 out]
                n2685 = flat-sequence {
                  tunnel: w6606 -> [w6611]
                  tunnel: w6605 -> [w6610]
                  tunnel: [w6611] -> w6602
                  tunnel: [w6610] -> w6601
                  tunnel: w6602 -> [w6616]
                  tunnel: w6601 -> [w6615]
                  frame #0 {
                    n2686 = local write "ROIXOffset"(w6611) -> ()
                    n2687 = local write "ROIYOffset"(w6610) -> ()
                  }
                  frame #1 {
                    n2688 = local read "Binning"() -> (w6637:u16)
                    n2689 = local read "ROIWidth"() -> (w6630:u16)
                    n2690 = local read "ROIHeight"() -> (w6631:u16)
                    n2691 = local read "Naxis1"() -> (w6635:u16)
                    n2692 = local read "Naxis2"() -> (w6634:u16)
                    n2693 = local read "XROIRef"() -> (w6628:dbl)
                    n2694 = local read "YROIRef"() -> (w6614:dbl)
                    n2695 = Bundle("ROIXOffset"=w6616, "ROIYOffset"=w6615) -> (w6632:cluster{"ROIXOffset":u16, "ROIYOffset":u16})  [unwired: 1 in]
                    n2696 = Bundle("Naxis1"=w6635, "Naxis2"=w6634) -> (w6636:cluster{"Naxis1":u16, "Naxis2":u16})  [unwired: 1 in]
                    n2697 = Bundle("ROIWidth"=w6630, "ROIHeight"=w6631) -> (w6633:cluster{"ROIWidth":u16, "ROIHeight":u16})  [unwired: 1 in]
                    n2698 = Bundle("XROIRef"=w6628, "YROIRef"=w6614) -> (w6629:cluster{"XROIRef":dbl, "YROIRef":dbl})  [unwired: 1 in]
                    n2699 = call "SAOMM-ROI_Fixer.vi"("Binning"=w6637, "Use Offset?"=TRUE, "naxis"=w6636, "ROI"=w6633, "Offset"=w6632, "Reference Pixel"=w6629) -> ("FixedOffset"=w6619:cluster{"ROIXOffset":u16, "ROIYOffset":u16}, "FixedPixel"=w6617:cluster{"PixelX":dbl, "PixelY":dbl})  [unwired: 6 in, 2 out]
                    n2700 = Unbundle By Name(w6619) -> ("ROIXOffset"=w6627:u16, "ROIYOffset"=w6626:u16)
                    n2701 = local read "MessageType"() -> (w6639:cluster{string[], u32[]})
                    n2702 = control-ref of="PrAMS-ACK"() -> (w6640:refnum<vi>)
                    n2703 = control-ref of="PrAMS actif"() -> (w6645:refnum<vi>)
                    n2704 = local read "PrAMS VRN"() -> (w6644:refnum<visa-resource-name>)
                    n2705 = local read "PrAMS Error"() -> (w6643:errorcluster)
                    n2706 = Unbundle By Name(w6617) -> ("PixelX"=w6620:dbl, "PixelY"=w6623:dbl)
                    n2707 = To Double Precision Float(number=w6627) -> (double precision float=w6622:dbl)
                    n2708 = To Double Precision Float(number=w6626) -> (double precision float=w6621:dbl)
                    n2709 = Bundle("ROIYOffset"=w6626, "ROIXOffset"=w6627) -> (w6618:cluster{"ROIYOffset":u16, "ROIXOffset":u16})  [unwired: 1 in]
                    n2710 = Add(x=w6621, y=w6620) -> (x+y=w6613:dbl)
                    n2711 = Add(x=w6622, y=w6623) -> (x+y=w6612:dbl)
                    n2712 = call "SAOMM-UpdateROI.vi"("PRAMMS-COMM IN"=w6644, "Active Refnum"=w6645, "PrAMS-ACK"=w6640, "MessageType"=w6639, "Error IN"=w6643, "Position"=w6618) -> ("PRAMMS-COMM OUT"=w6642:refnum<visa-resource-name>, "Error OUT"=w6641:errorcluster)  [unwired: 7 in, 1 out]
                    n2713 = property on="ImgArray" class="IntGraph (strict)"() -> ("Cursor.Cursor Position"=w6625:T44)  [unwired: 2 in, 2 out]
                    n2714 = local write "XReference"(w6613) -> ()
                    n2715 = local write "YReference"(w6612) -> ()
                    n2716 = local write "PrAMS Error"(w6641) -> ()
                    n2717 = local write "PrAMS VRN"(w6642) -> ()
                    n2718 = Bundle(cluster=w6625, "Cursor X"=w6613, "Cursor Y"=w6612) -> (w6624:T44)
                    n2719 = property on="ImgArray" class="IntGraph (strict)"("Cursor.Cursor Position"=w6624) -> ()  [unwired: 2 in, 2 out]
                  }
                }
              }
              event "go Ouest", "go Nord", "go Est", "go Sud": Mouse Down {
                n2720 = event-data() -> ()  [unwired: 1 in, 8 out]
                n2721 = Compound Arithmetic op=OR("go Nord", "go Sud", "go Est", "go Ouest") -> (w6646:bool)
                n2722 = local write "enfoncé"(w6646) -> ()
                n2723 = case shown="True" w6646 {
                  tunnel: "go Nord" -> [_ w6655]
                  tunnel: "go Sud" -> [_ w6654]
                  tunnel: "go Est" -> [_ w6653]
                  tunnel: "go Ouest" -> [_ w6652]
                  frame False {
                  }
                  frame True {
                    n2724 = local read "act_sonde"() -> (w6651:bool)
                    n2725 = Build Array(w6655, w6654, w6653, w6652) -> (w6657:bool[])
                    n2726 = Boolean Array To Number(Boolean array=w6657) -> (number=w6656:u32)
                    n2727 = case shown="True" w6651 {
                      tunnel: w6656 -> [w6663 w6720]
                      frame False {
                        # "0.1=1'/sec"
                        n2728 = local read "FieldAstrom"() -> (w6661:T4)
                        n2729 = local read "ImgAstrom"() -> (w6660:T4)
                        n2730 = while {
                          tunnel: w6663 -> [w6681]
                          tunnel: 0.1 ("t") -> [w6678]
                          tunnel: w6661 -> [w6672]
                          tunnel: w6660 -> [w6675]
                          tunnel: [FALSE] -> w6659
                          tunnel: u32 0 ("Active Cursor") -> [w6664]
                          stop <- w6676 continue-if-true
                          n2731 = property on="TableXYPos" class="XYGraph (strict)"("Active Cursor"=w6664) -> (error out=w6668:errorcluster)  [unwired: 2 in, 1 out]
                          n2732 = property on="TableXYPos" class="XYGraph (strict)"(error in=w6668) -> (error out=w6666:errorcluster, "Cursor.Cursor Position"=w6667:T44)  [unwired: 1 in, 1 out]
                          n2733 = Unbundle(w6667) -> ("Cursor X"=w6680:dbl, "Cursor Y"=w6679:dbl)
                          n2734 = case shown="0, Default" w6681 {
                            tunnel: [w6703 w6704 w6708 w6713 w6717] -> w6673
                            tunnel: w6680 -> [w6703 w6704 w6708 w6715 w6719]
                            tunnel: [w6702 w6705 w6710 w6712 w6718] -> w6674
                            tunnel: w6679 -> [w6702 w6707 w6709 w6712 w6718]
                            tunnel: w6678 -> [_ w6706 w6711 w6714 w6716]
                            frame 0, Default {
                            }
                            frame 1 {
                              n2735 = Add(x=w6707, y=w6706) -> (x+y=w6705:dbl)
                            }
                            frame 2 {
                              n2736 = Subtract(x=w6709, y=w6711) -> (x-y=w6710:dbl)
                            }
                            frame 4 {
                              n2737 = Add(x=w6715, y=w6714) -> (x+y=w6713:dbl)
                            }
                            frame 8 {
                              n2738 = Subtract(x=w6719, y=w6716) -> (x-y=w6717:dbl)
                            }
                          }
                          n2739 = Wait (ms)(milliseconds to wait=u32 100) -> ()  [unwired: 1 out]
                          n2740 = Bundle("Cursor X"=w6673, "Cursor Y"=w6674) -> (w6682:cluster{"Cursor X":dbl, "Cursor Y":dbl})  [unwired: 1 in]
                          n2741 = property on="TableXYPos" class="XYGraph (strict)"(error in=w6666, "Cursor.Cursor Position"=w6682) -> ()  [unwired: 1 in, 2 out]
                          n2742 = call "xy2ad.vi"("Y (px)"=w6674, "X (px)"=w6673, "Astrometry"=w6672) -> ("DEC (°)"=w6670:dbl, "RA (°)"=w6671:dbl)  [unwired: 5 in, 2 out]
                          n2743 = local read "ImageDSSLed"() -> (w6665:bool)
                          n2744 = case shown="True" w6665 {
                            tunnel: w6675 -> [_ w6691]
                            tunnel: w6671 -> [_ w6690]
                            tunnel: w6670 -> [_ w6689]
                            frame False {
                            }
                            frame True {
                              w6687 = u16 1 items=["Region d'intérêt", "Prévisualisation", "Idle"] ("ImageUsage")
                              n2745 = call "ad2xy.vi"("DEC"=w6689, "RA"=w6690, "Astrometry"=w6691) -> ("Y"=w6693:dbl, "X"=w6694:dbl)  [unwired: 6 in, 1 out]
                              n2746 = local read "ImgData"() -> (w6699:sgl[][])
                              n2747 = To Long Integer(number=w6694) -> (32bit integer=w6697:i32)
                              n2748 = To Long Integer(number=w6693) -> (32bit integer=w6698:i32)
                              n2749 = call "subimage.vi"("Ysz/2"=100 ("Xsz/2"), "Xsz/2"=100, "Yc"=w6698, "Xc"=w6697, "ImgData"=w6699) -> ("SubImg"=w6700:sgl[][])  [unwired: 6 in]
                              n2750 = local write "SubIMG4DSS?"(TRUE ("SubIMG4DSS?")) -> ()
                              n2751 = Array Max & Min(array=w6700) -> (max value=w6701:sgl)  [unwired: 3 out]
                              n2752 = local write "ImageUsage"(w6687) -> ()
                              n2753 = call "Draw_crosshair.vi"("Image IN"=w6700, "White Value"=w6701) -> ("Image OUT"=w6692:sgl[][])  [unwired: 13 in]
                              n2754 = local write "subimg"(w6692) -> ()
                            }
                          }
                          n2755 = local read "go Nord"() -> (w6684:bool)
                          n2756 = local read "go Ouest"() -> (w6686:bool)
                          n2757 = local read "go Est"() -> (w6685:bool)
                          n2758 = local read "go Sud"() -> (w6683:bool)
                          n2759 = Compound Arithmetic op=OR(w6686, w6685, w6684, w6683) -> (w6676:bool)
                          n2760 = local write "enfoncé"(w6676) -> ()
                        }
                        n2761 = local write "go Nord"(w6659) -> ()
                        n2762 = local write "go Ouest"(w6659) -> ()
                        n2763 = local write "go Est"(w6659) -> ()
                        n2764 = local write "go Sud"(w6659) -> ()
                        n2765 = local write "enfoncé"(w6659) -> ()
                      }
                      frame True {
                        n2766 = flat-sequence {
                          tunnel: w6720 -> [w6722]
                          frame #0 {
                            # "Vrai = buggy continuous\nFaux = nouveau pas-à-pas"
                            n2767 = case shown="True" FALSE {
                              tunnel: w6722 -> [w6724 w6767]
                              frame False {
                                n2768 = flat-sequence {
                                tunnel: w6724 -> [w6726]
                                tunnel: [w6726] -> w6723
                                tunnel: w6723 -> [w6743]
                                frame #0 {
                                w6725 = FALSE ("go Ouest")
                                n2769 = local write "go Nord"(w6725) -> ()
                                n2770 = local write "go Ouest"(w6725) -> ()
                                n2771 = local write "go Est"(w6725) -> ()
                                n2772 = local write "go Sud"(w6725) -> ()
                                n2773 = local write "enfoncé"(w6725) -> ()
                                }
                                frame #1 {
                                # "Devrait être remplacé par la valeur théorique ..."
                                n2774 = property on="TableXYPos" class="XYGraph (strict)"("Active Cursor"=u32 1) -> (error out=w6746:errorcluster)  [unwired: 2 in, 1 out]
                                n2775 = property on="TableXYPos" class="XYGraph (strict)"(error in=w6746) -> ("Cursor.Cursor Position"=w6744:T44)  [unwired: 1 in, 2 out]
                                n2776 = Unbundle(w6744) -> ("Cursor X"=w6748:dbl, "Cursor Y"=w6747:dbl)
                                n2777 = case shown="1" w6743 {
                                tunnel: [w6750 w6751 w6755 w6760 w6764] -> w6741
                                tunnel: w6748 -> [w6750 w6751 w6755 w6762 w6766]
                                tunnel: [w6749 w6752 w6757 w6759 w6765] -> w6740
                                tunnel: w6747 -> [w6749 w6754 w6756 w6759 w6765]
                                tunnel: "ClickJOG" -> [_ w6753 w6758 w6761 w6763]
                                frame 0, Default {
                                }
                                frame 1 {
                                n2778 = Add(x=w6754, y=w6753) -> (x+y=w6752:dbl)
                                }
                                frame 2 {
                                n2779 = Subtract(x=w6756, y=w6758) -> (x-y=w6757:dbl)
                                }
                                frame 4 {
                                n2780 = Add(x=w6762, y=w6761) -> (x+y=w6760:dbl)
                                }
                                frame 8 {
                                n2781 = Subtract(x=w6766, y=w6763) -> (x-y=w6764:dbl)
                                }
                                }
                                n2782 = local read "FieldAstrom"() -> (w6739:T4)
                                n2783 = call "xy2ad.vi"("Y (px)"=w6740, "X (px)"=w6741, "Astrometry"=w6739) -> ("DEC (°)"=w6737:dbl, "RA (°)"=w6738:dbl)  [unwired: 5 in, 2 out]
                                n2784 = local read "Position Z"() -> (w6733:dbl)
                                n2785 = local read "TableAstrom"() -> (w6736:T4)
